vi "2D_interpolation.vi"(0 "X Axis Current":dbl[](array[numeric])=[-740.0, -570.0, -450.0, -340.0, -240.0, -150.0, -90.0, -30.0, 30.0, 90.0, 150.0, 240.0, 340.0, 450.0, 570.0, 740.0] format="%.2f", 1 "Min Z Value In":dbl format="%.2f", 5 "Y axis Current":dbl[](array[numeric])=[0.0, 1.0, 2.0, 3.0, 4.0] format="%.2f", 7 "Bkgnd Value":dbl, 9 "Plot In":dbl[][](graph)=[[0.00729, 0.1932, 1.451, 8.716, 18.11, 23.03, 24.73, 25.78, 25.44, 25.13, 24.23, 19.22, 10.83, 2.468, 0.2041, 0.06197], [0.04411, 0.08454, 1.327, 8.642, 17.93, 24.19, 25.23, 26.19, 26.05, 25.99, 24.99, 18.91, 9.149, 2.415, 0.2169, 0.07351], [0.05478, 0.1242, 1.515, 6.946, 14.88, 20.98, 22.81, 24.04, 24.28, 23.16, 20.91, 14.16, 6.61, 1.632, 0.1789, 0.1022], [0.04013, 0.1423, 1.178, 4.932, 9.291, 12.85, 15.3, 17.51, 17.21, 15.68, 12.8, 8.551, 4.232, 1.222, 0.1313, 0.08755], [0.04404, 0.1138, 0.7891, 2.319, 4.114, 6.265, 7.369, 8.39, 7.964, 7.127, 5.656, 3.956, 2.019, 0.6129, 0.1615, 0.08441]], 11 "Increment Value":dbl=1.0 format="%.2f", 12 "Transpose":bool=TRUE, 13 "Point Size":i32) -> (2 "min Z value":dbl format="%.2f", 3 "max Z value":dbl format="%.2f", 8 "Increment Value Out":dbl, 14 "Plot Out":dbl[][](graph)=[[0.00729, 0.18153463174730816, 0.17352738437348433, 1.6752433719500537, 8.231465735195274, 17.570357598383207, 23.099772817121426, 25.58386930448374, 25.31727725753219, 24.28926231541072, 18.717383219374323, 10.355253339797807, 2.7760273383248344, 0.3109897541921306, 0.08276881403435009, 0.06197], [0.04411, 0.1361526368018142, 0.04039202183336771, 1.5611636795339547, 8.176972694107874, 17.32000974741714, 24.257541358764026, 25.949153465972987, 26.01802540761648, 25.060373307424115, 18.284750328365213, 8.689831176707928, 2.642937641487066, 0.43219350072447926, -0.019957690739617468, 0.07351], [0.05478, 0.03446320268089581, 0.2086595806581808, 1.6919212249796047, 6.580368005180591, 14.333585185483123, 21.06810094963999, 23.709254571137723, 24.04768940379576, 21.01660820522005, 13.60443428327954, 6.2766496258038735, 1.7988963349022484, 0.2952877651784204, 0.05436788410934033, 0.1022], [0.04013, 0.06419557464541133, 0.2035068586120256, 1.3118741659450193, 4.7061387064566835, 9.009825946069038, 12.927700276268434, 17.003135081884164, 16.83885730812343, 12.902263313363814, 8.246161922417906, 4.035269404379355, 1.329605659745338, 0.24574055091433544, 0.012829784119986217, 0.08755], [0.04404, 0.022691144295571734, 0.19102098261858932, 0.8525411026079828, 2.2353542219792946, 3.966676465246214, 6.305347763088489, 8.17672908183636, 7.7348668140659, 5.703994479070454, 3.8329088824353237, 1.9256956625267279, 0.6611488869641811, 0.20508248283573002, 0.10119553469307395, 0.08441]])   [LabVIEW 2010]
uses:
  Results_plotter_Global.vi
  <vilib>/Analysis/NI_AALPro.lvlib
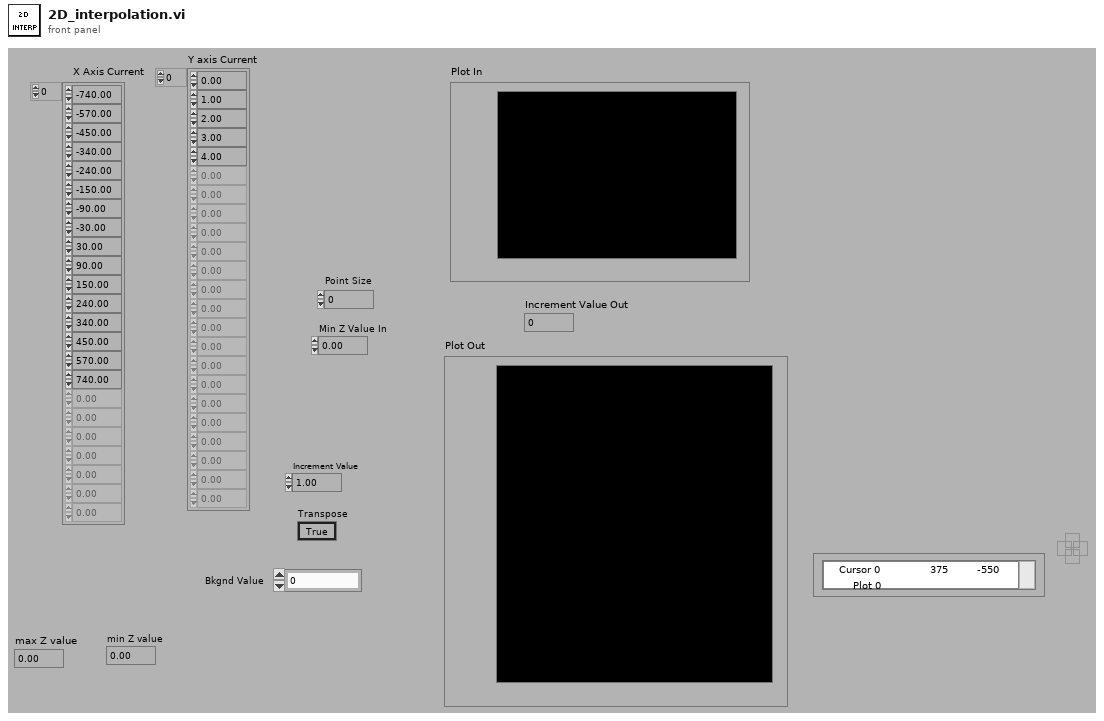
[diagram p1: front panel]
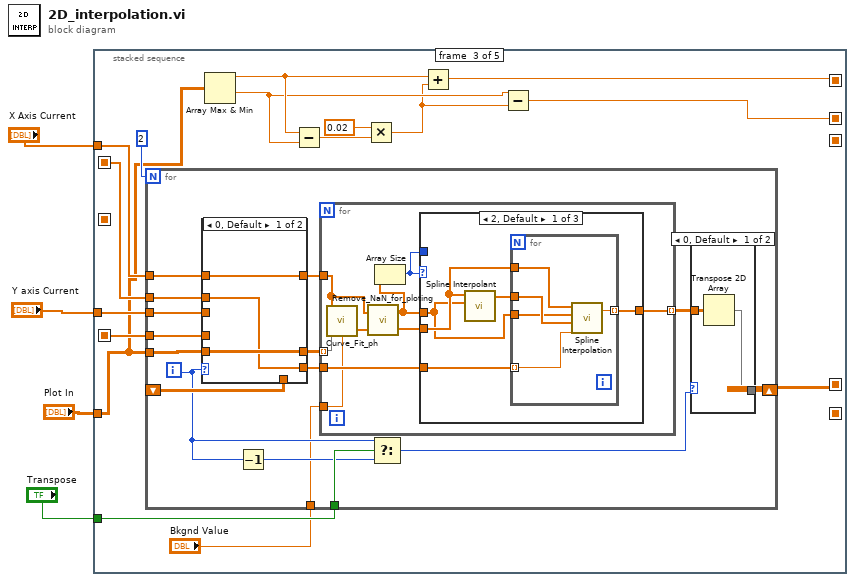
[diagram p0: block diagram]
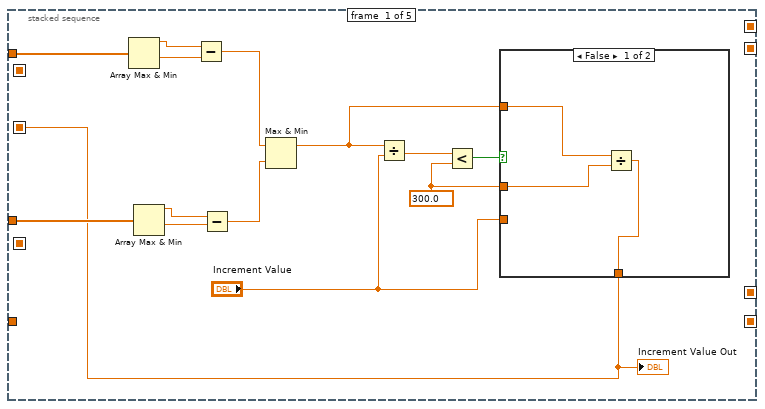
[diagram p2: hidden frame]
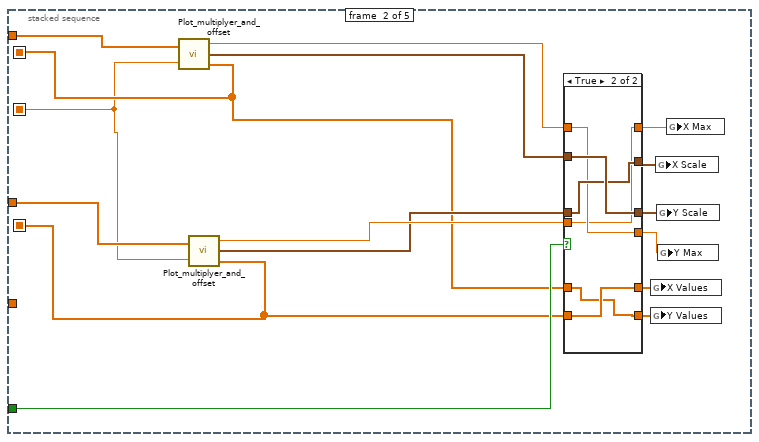
[diagram p4: hidden frame]
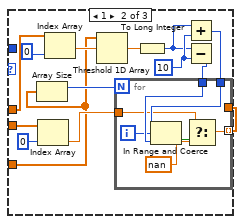
[diagram p8: hidden frame]
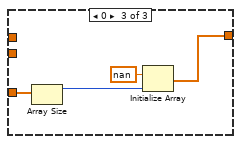
[diagram p9: hidden frame]
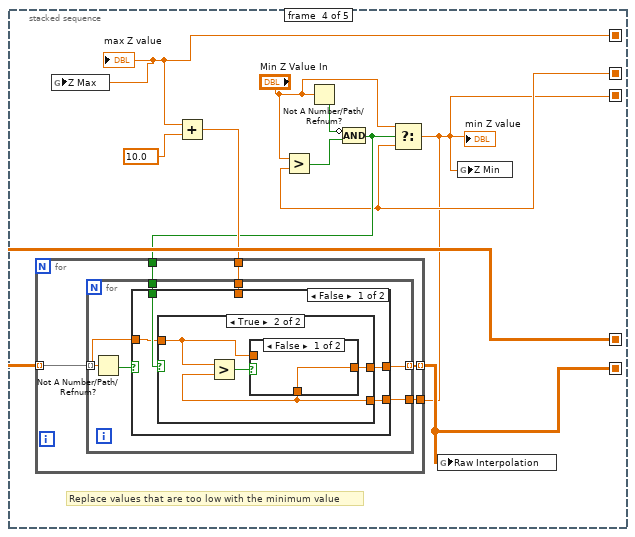
[diagram p10: hidden frame]
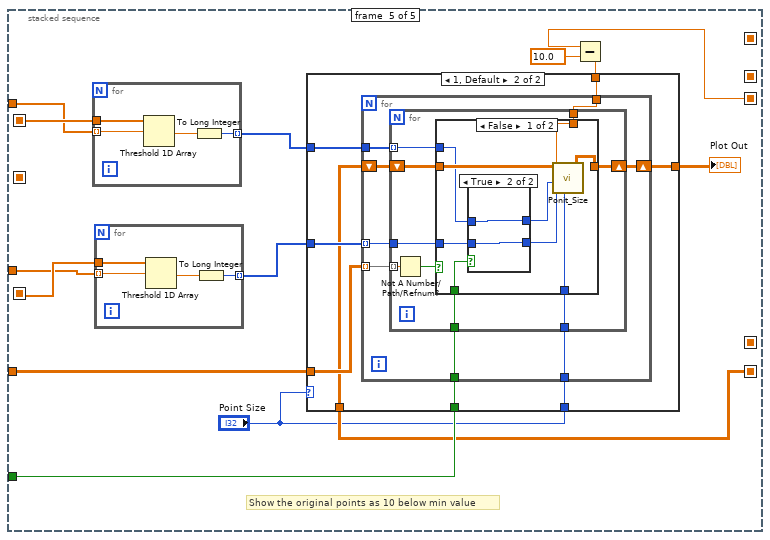
[diagram p14: hidden frame]
diagram:
  n1 = stacked-sequence {
    seq-local: [_ w27 _ _ _] -> [_ _ w64 _ w183]
    seq-local: [_ w25 _ _ _] -> [_ _ w62 _ w181]
    seq-local: [_ _ w60 _ _] -> [_ _ _ w146 _]
    seq-local: [_ _ w55 _ _] -> [_ _ _ w136 _]
    seq-local: [_ _ w52 _ _] -> [_ _ _ w139 _]
    seq-local: [_ _ _ w138 _] -> [_ _ _ _ w171]
    seq-local: [_ _ _ w137 _] -> [_ _ _ _ w172]
    seq-local: [w8 _ _ _ _] -> [_ w23 _ _ _]
    tunnel: "X Axis Current" -> [w18 w37 w65 _ w182]
    tunnel: "Y axis Current" -> [w17 w34 w63 _ w180]
    tunnel: "Transpose" -> [_ w38 w61 _ w176]
    tunnel: "Plot In" -> [_ _ w59 _ w179]
    frame #0 {
      w5 = 300.0 ("y")
      n2 = Array Max & Min(array=w18) -> (max value=w16:dbl, min value=w15:dbl)  [unwired: 2 out]
      n3 = Array Max & Min(array=w17) -> (max value=w14:dbl, min value=w13:dbl)  [unwired: 2 out]
      n4 = Subtract(x=w16, y=w15) -> (x-y=w11:dbl)
      n5 = Subtract(x=w14, y=w13) -> (x-y=w12:dbl)
      n6 = Max & Min(x=w11, y=w12) -> (max(x,y)=w6:dbl)  [unwired: 1 out]
      n7 = Divide(x=w6, y="Increment Value") -> (x/y=w10:dbl)
      n8 = Less?(x=w10, y=w5) -> (x < y?=w9:bool)
      n9 = case shown="False" w9 {
        tunnel: [w19 w22] -> w8
        tunnel: "Increment Value" -> [_ w22]
        tunnel: w6 -> [w21 _]
        tunnel: w5 -> [w20 _]
        frame False {
          n10 = Divide(x=w21, y=w20) -> (x/y=w19:dbl)
        }
        frame True {
        }
      }
      "Increment Value Out" <- w8
    }
    frame #1 {
      n11 = call "Plot_multiplyer_and_offset.vi"("Position in"=w37, "Increment Value"=w23) -> ("Max Value"=w35:dbl, "Scale"=w36:cluster{"Xo":dbl, "delta X":dbl}, "Position Out"=w27:dbl[])
      n12 = call "Plot_multiplyer_and_offset.vi"("Position in"=w34, "Increment Value"=w23) -> ("Max Value"=w33:dbl, "Scale"=w32:cluster{"Xo":dbl, "delta X":dbl}, "Position Out"=w25:dbl[])
      n13 = case shown="True" w38 {
        tunnel: [w44 w49] -> w30
        tunnel: w36 -> [w44 w50]
        tunnel: [w43 w50] -> w31
        tunnel: w32 -> [w43 w49]
        tunnel: [w42 w47] -> w28
        tunnel: w35 -> [w42 w48]
        tunnel: [w41 w48] -> w29
        tunnel: w33 -> [w41 w47]
        tunnel: w27 -> [w40 w45]
        tunnel: [w40 w46] -> w26
        tunnel: w25 -> [w39 w46]
        tunnel: [w39 w45] -> w24
        frame False {
        }
        frame True {
        }
      }
      n14 = global write "Results_plotter_Global.vi" "X Values"(w26) -> ()
      n15 = global write "Results_plotter_Global.vi" "Y Values"(w24) -> ()
      n16 = global write "Results_plotter_Global.vi" "X Scale"(w30) -> ()
      n17 = global write "Results_plotter_Global.vi" "Y Scale"(w31) -> ()
      n18 = global write "Results_plotter_Global.vi" "Y Max"(w29) -> ()
      n19 = global write "Results_plotter_Global.vi" "X Max"(w28) -> ()
    }
    frame #2 {
      n20 = for {
        N: 2 -> [_]
        tunnel: w59 -> [w81]
        shift-right: [w78] -> w60
        shift-left: _ -> [w79]
        tunnel: w65 -> [w75]
        tunnel: w64 -> [w74]
        tunnel: w63 -> [w73]
        tunnel: w62 -> [w72]
        tunnel: w61 -> [w71]
        tunnel: "Bkgnd Value" -> [w67]
        i -> [w68]
        n21 = case shown="0, Default" w68 {
          tunnel: w81 -> [w88 _]
          tunnel: [w88 w91] -> w80
          tunnel: w79 -> [_ w91]
          tunnel: [w87 w90] -> w77
          tunnel: [w86 w89] -> w76
          tunnel: w75 -> [w87 _]
          tunnel: w74 -> [w86 _]
          tunnel: w73 -> [_ w90]
          tunnel: w72 -> [_ w89]
          frame 0, Default {
          }
          frame 1 {
          }
        }
        n22 = Decrement(x=w68) -> (x-1=w69:i32)
        n23 = for {
          tunnel: w80 -> [w95] mode=indexing
          tunnel: w77 -> [w93]
          tunnel: [w100] -> w82 mode=indexing
          tunnel: w76 -> [w99]
          tunnel: w67 -> [w92]
          n24 = call "Curve_Fit_ph.vi"("Bkgnd Value"=w92, "Values In"=w95, "Positions"=w93) -> ("Values Out"=w94:dbl[])  [unwired: 1 in, 1 out]
          n25 = call "Remove_NaN_for_ploting.vi"("Array 2"=w94, "Array 1"=w93) -> ("Array 2 Out"=w98:dbl[], "Array 1 Out"=w97:dbl[])
          n26 = Array Size(array=w97) -> (size(s)=w96:i32)
          n27 = case shown="2, Default" w96 {
            tunnel: [w104 w118 w135] -> w100
            tunnel: w99 -> [w103 w111 w133]
            tunnel: w98 -> [w102 w112 _]
            tunnel: w97 -> [w101 w122 _]
            tunnel: w96 -> [_ _ _]
            frame 2, Default {
              n28 = call <vilib>:"Spline Interpolant.vi"("X"=w101, "Y"=w102) -> ("Interpolant"=w105:dbl[])  [unwired: 2 in, 1 out]
              n29 = for {
                tunnel: w105 -> [w110]
                tunnel: w102 -> [w109]
                tunnel: w101 -> [w108]
                tunnel: [w107] -> w104 mode=indexing
                tunnel: w103 -> [w106] mode=indexing
                n30 = call <vilib>:"Spline Interpolation.vi"("x value"=w106, "Interpolant"=w110, "X"=w108, "Y"=w109) -> ("interpolation value"=w107:dbl)  [unwired: 1 out]
              }
            }
            frame 1 {
              w115 = 10 ("y")
              n31 = Array Size(array=w111) -> (size(s)=w113:i32)
              n32 = Index Array(array=w112, index=0 ("Index")) -> (element=w117:dbl)
              n33 = Index Array(array=w122, index=0 ("Index")) -> (element=w116:dbl)
              n34 = Threshold 1D Array(2:w116, 3:w111) -> (0:w121:dbl)  [unwired: 1 out]
              n35 = To Long Integer(number=w121) -> (32bit integer=w114:i32)
              n36 = Add(x=w114, y=w115) -> (x+y=w120:i32)
              n37 = Subtract(x=w114, y=w115) -> (x-y=w119:i32)
              n38 = for {
                N: w113 -> [_]
                tunnel: w120 -> [w131]
                tunnel: w119 -> [w130]
                tunnel: [w128] -> w118 mode=indexing
                tunnel: w117 -> [w127]
                i -> [w125]
                n39 = In Range and Coerce(upper limit=w131, x=w125, lower limit=w130) -> (In Range?=w129:bool)  [unwired: 1 out]
                n40 = Select(t=w127, s=w129, f=nan) -> (s? t:f=w128:dbl)
              }
            }
            frame 0 {
              n41 = Array Size(array=w133) -> (size(s)=w132:i32)
              n42 = Initialize Array(nan ("Element Data"), w132) -> (w135:dbl[])
            }
          }
        }
        n43 = Select(t=w68, s=w71, f=w69) -> (s? t:f=w70:i32)
        n44 = case shown="0, Default" w70 {
          tunnel: w82 -> [w84 w85]
          tunnel: [w83 w85] -> w78
          frame 0, Default {
            n45 = Transpose 2D Array(2D array=w84) -> (transposed array=w83:dbl[][])
          }
          frame 1 {
          }
        }
      }
      n46 = Array Max & Min(array=w59) -> (max value=w56:dbl, min value=w54:dbl)  [unwired: 2 out]
      n47 = Subtract(x=w56, y=w54) -> (x-y=w58:dbl)
      n48 = Multiply(x=0.02, y=w58) -> (x*y=w53:dbl)
      n49 = Add(x=w56, y=w53) -> (x+y=w55:dbl)
      n50 = Subtract(x=w54, y=w53) -> (x-y=w52:dbl)
    }
    frame #3 {
      # "Replace values that are too low with the minimum value"
      n51 = global write "Results_plotter_Global.vi" "Z Max"(w136) -> ()
      n52 = Add(x=w136, y=10.0) -> (x+y=w144:dbl)
      n53 = Greater?(x="Min Z Value In", y=w139) -> (0:w143:bool)
      n54 = Not A Number/Path/Refnum?(number/path/refnum="Min Z Value In") -> (NaN/Path/Refnum?=w142:bool)
      n55 = Compound Arithmetic op=AND(invert w142, w143) -> (w140:bool)
      n56 = Select(t="Min Z Value In", s=w140, f=w139) -> (s? t:f=w137:dbl)
      "min Z value" <- w137
      n57 = for {
        tunnel: w146 -> [w151] mode=indexing
        tunnel: w144 -> [w150]
        tunnel: [w149] -> w138 mode=indexing
        tunnel: w140 -> [w148]
        tunnel: w137 -> [w147]
        n58 = for {
          tunnel: w151 -> [w153] mode=indexing
          tunnel: w150 -> [w155]
          tunnel: [w156] -> w149 mode=indexing
          tunnel: w148 -> [w154]
          tunnel: w147 -> [w152]
          n59 = Not A Number/Path/Refnum?(number/path/refnum=w153) -> (NaN/Path/Refnum?=w157:bool)
          n60 = case shown="False" w157 {
            tunnel: [w158 w169] -> w156
            tunnel: w155 -> [_ w169]
            tunnel: w154 -> [w161 _]
            tunnel: w153 -> [w160 _]
            tunnel: w152 -> [w159 _]
            frame False {
              n61 = case shown="True" w161 {
                tunnel: w160 -> [w162 w164]
                tunnel: w159 -> [_ w163]
                tunnel: [w162 w165] -> w158
                frame False {
                }
                frame True {
                  n62 = Greater?(x=w164, y=w163) -> (0:w166:bool)
                  n63 = case shown="False" w166 {
                    tunnel: [w167 w168] -> w165
                    tunnel: w164 -> [_ w168]
                    tunnel: w163 -> [w167 _]
                    frame False {
                    }
                    frame True {
                    }
                  }
                }
              }
            }
            frame True {
            }
          }
        }
      }
      n64 = global write "Results_plotter_Global.vi" "Raw Interpolation"(w138) -> ()
      n65 = global write "Results_plotter_Global.vi" "Z Min"(w137) -> ()
      "max Z value" <- w136
    }
    frame #4 {
      # "Show the original points as 10 below min value"
      n66 = for {
        tunnel: w183 -> [w231]
        tunnel: w182 -> [w230] mode=indexing
        tunnel: [w228] -> w178 mode=indexing
        n67 = Threshold 1D Array(2:w230, 3:w231) -> (0:w229:dbl)  [unwired: 1 out]
        n68 = To Long Integer(number=w229) -> (32bit integer=w228:i32)
      }
      n69 = for {
        tunnel: w181 -> [w227]
        tunnel: w180 -> [w226] mode=indexing
        tunnel: [w224] -> w177 mode=indexing
        n70 = Threshold 1D Array(2:w226, 3:w227) -> (0:w225:dbl)  [unwired: 1 out]
        n71 = To Long Integer(number=w225) -> (32bit integer=w224:i32)
      }
      n72 = Subtract(x=w172, y=10.0) -> (x-y=w173:dbl)
      n73 = case shown="1, Default" "Point Size" {
        tunnel: w179 -> [_ w192]
        tunnel: w178 -> [_ w191]
        tunnel: w177 -> [_ w190]
        tunnel: w176 -> [_ w189]
        tunnel: [w184 w188] -> w175
        tunnel: w173 -> [_ w187]
        tunnel: w171 -> [w184 w186]
        tunnel: "Point Size" -> [_ w185]
        frame 0 {
        }
        frame 1, Default {
          n74 = for {
            tunnel: w192 -> [w200] mode=indexing
            shift-right: [w196] -> w188
            shift-left: w186 -> [w197]
            tunnel: w190 -> [w199] mode=indexing
            tunnel: w191 -> [w198]
            tunnel: w189 -> [w195]
            tunnel: w187 -> [w194]
            tunnel: w185 -> [w193]
            n75 = for {
              tunnel: w200 -> [w209] mode=indexing
              tunnel: w199 -> [w207]
              tunnel: w198 -> [w206] mode=indexing
              shift-right: [w205] -> w196
              shift-left: w197 -> [w204]
              tunnel: w195 -> [w203]
              tunnel: w194 -> [w202]
              tunnel: w193 -> [w201]
              n76 = Not A Number/Path/Refnum?(number/path/refnum=w209) -> (NaN/Path/Refnum?=w208:bool)
              n77 = case shown="False" w208 {
                tunnel: w207 -> [w213 _]
                tunnel: w206 -> [w212 _]
                tunnel: w204 -> [w218 w223]
                tunnel: [w217 w223] -> w205
                tunnel: w203 -> [w215 _]
                tunnel: w202 -> [w216 _]
                tunnel: w201 -> [w210 _]
                frame False {
                  n78 = case shown="True" w215 {
                    tunnel: [w220 w222] -> w214
                    tunnel: w213 -> [w219 w222]
                    tunnel: w212 -> [w220 w221]
                    tunnel: [w219 w221] -> w211
                    frame False {
                    }
                    frame True {
                    }
                  }
                  n79 = call "Ponit_Size.vi"("New Value"=w216, "Array In"=w218, "Index1"=w211, "Index2"=w214, "Size"=w210) -> ("Array Out"=w217:dbl[][])
                }
                frame True {
                }
              }
            }
          }
        }
      }
      "Plot Out" <- w175
    }
  }
